vi "Dilution_visibleRed.vi"(4 "calculated":u16, 6 "dilution":bool) -> (0 "MFC3":u16(ring)=2 items=["Enabled", "Disabled", "Disabled and Grayed Out"], 1 "MFC2":u16(ring)=2 items=["Enabled", "Disabled", "Disabled and Grayed Out"], 2 "MFC1":u16(ring)=2 items=["Enabled", "Disabled", "Disabled and Grayed Out"], 3 "flow":u16(ring)=2 items=["Enabled", "Disabled", "Disabled and Grayed Out"])   [LabVIEW 2011]
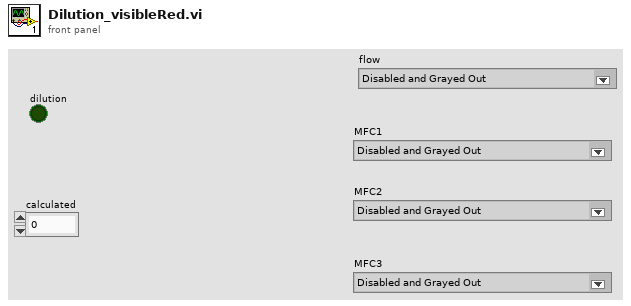
[diagram p1: front panel]
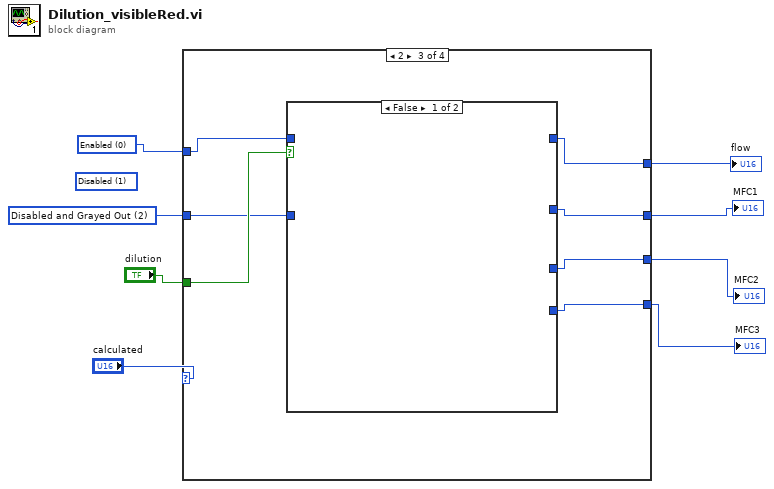
[diagram p0: block diagram]
diagram:
  w4 = u16 2 items=["Enabled", "Disabled", "Disabled and Grayed Out"] ("flow 2")
  (unwired) u16 1 items=["Enabled", "Disabled", "Disabled and Grayed Out"] ("flow 2")
  w5 = u16 0 items=["Enabled", "Disabled", "Disabled and Grayed Out"] ("flow 2")
  n1 = case shown="2" "calculated" {
    tunnel: "dilution" -> [w15 w26 w37 w46]
    tunnel: [w9 w23 w35 w44] -> w6
    tunnel: w5 -> [w14 w25 w36 w45]
    tunnel: w4 -> [w13 w24 w32 w41]
    tunnel: [w12 w21 w33 w40] -> w3
    tunnel: [w11 w20 w34 w43] -> w2
    tunnel: [w10 w22 w31 w42] -> w1
    frame 0, Default {
      n2 = case shown="True" w15 {
        tunnel: w14 -> [w16 w19]
        tunnel: [w17 w18] -> w9
        tunnel: w13 -> [w17 w18]
        tunnel: [_ w19] -> w12
        tunnel: [w16 w19] -> w11
        tunnel: [_ w19] -> w10
        frame False {
        }
        frame True {
        }
      }
    }
    frame 1 {
      n3 = case shown="True" w26 {
        tunnel: w25 -> [w28 w30]
        tunnel: w24 -> [w27 w29]
        tunnel: [w28 w30] -> w23
        tunnel: [_ w30] -> w22
        tunnel: [_ w30] -> w21
        tunnel: [w27 w29] -> w20
        frame False {
        }
        frame True {
        }
      }
    }
    frame 2 {
      n4 = case shown="False" w37 {
        tunnel: w36 -> [_ w39]
        tunnel: [_ w39] -> w35
        tunnel: [_ w39] -> w34
        tunnel: [_ w39] -> w33
        tunnel: w32 -> [_ w38]
        tunnel: [_ w38] -> w31
        frame False {
        }
        frame True {
        }
      }
    }
    frame 3 {
      n5 = case shown="True" w46 {
        tunnel: w45 -> [_ w48]
        tunnel: [_ w48] -> w44
        tunnel: [_ w48] -> w43
        tunnel: [_ w48] -> w42
        tunnel: [_ w47] -> w40
        tunnel: w41 -> [_ w47]
        frame False {
        }
        frame True {
        }
      }
    }
  }
  "flow" <- w6
  "MFC1" <- w2
  "MFC2" <- w1
  "MFC3" <- w3
